vi "manageDependenciesScript.vi"() -> ()   [LabVIEW 2016]
panel:
  out "size(s)":i32
  out "Dependency Paths":path[](array[path])
  out "Dependency Names":string[](array[string])
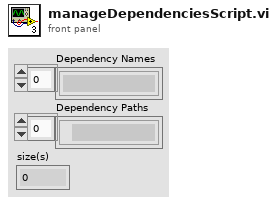
[diagram p1: front panel]
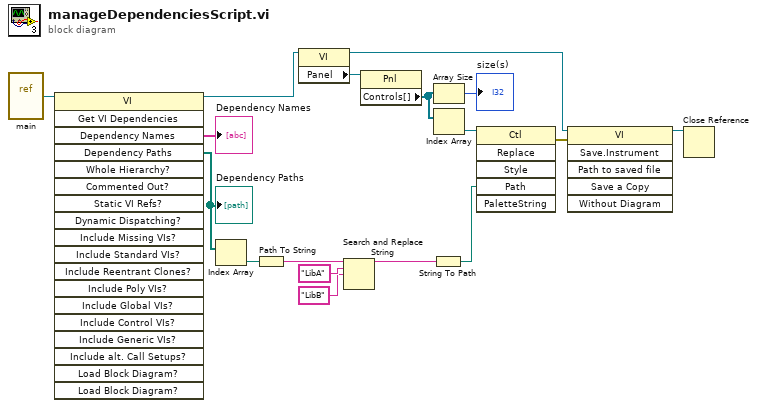
[diagram p0: block diagram]
diagram:
  n1 = vi-ref "main.vi"() -> (w17:refnum<vi>)
  n2 = invoke class="VI" method="Get VI Dependencies"(reference=w17) -> (reference out=w15:refnum<vi>, "Dependency Names"=→"Dependency Names":string[], "Dependency Paths"=w10:path[])  [unwired: 18 in, 16 out]
  "Dependency Paths" <- w10
  n3 = Index Array(array=w10) -> (element=w9:path)  [unwired: 1 in]
  n4 = Path To String(path=w9) -> (string=w8:string)
  n5 = property class="VI"(reference=w15) -> (reference out=w3:refnum<vi>, "Panel"=w14:refnum<vi>)  [unwired: 1 in, 1 out]
  n6 = Search and Replace String(input string=w8, search string="LibA" ("substring (\"\")"), replace string="LibB" ("replace string (\"\")")) -> (result string=w5:string)  [unwired: 5 in, 3 out]
  n7 = property class="Pnl"(reference=w14) -> ("Controls[]"=w12:refnum<vi>[])  [unwired: 1 in, 2 out]
  n8 = String To Path(string=w5) -> (path=w4:path)
  n9 = Array Size(array=w12) -> (size(s)=→"size(s)":i32)
  n10 = Index Array(array=w12) -> (element=w11:refnum<vi>)  [unwired: 1 in]
  n11 = invoke class="Ctl" method="Replace"(reference=w11, "Path"=w4) -> (error out=w1:errorcluster)  [unwired: 4 in, 5 out]
  n12 = invoke class="VI" method="Save.Instrument"(reference=w3, error in=w1) -> (reference out=w2:refnum<vi>)  [unwired: 4 in, 5 out]
  n13 = Close Reference(reference=w2) -> ()  [unwired: 1 in, 1 out]
